vi "Configure Probe.vi"   [LabVIEW 2016, in "Tektronix DPO MSO 2000 4000 Series.lvlib"]
doc: "Select an input type for an oscilloscope and configures the probe settings. The available input types includes:\nAuxiliary Input\nChannel Input"
uses:
  Tektronix DPO MSO 2000 4000 Series.lvlib
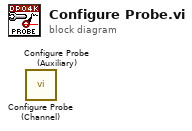
[diagram p0: block diagram]
diagram:
  n1 = call "Configure Probe (Channel).vi"() -> ()  [unwired: 10 in, 2 out]
  n2 = call "Configure Probe (Auxiliary).vi"() -> ()  [unwired: 10 in, 2 out]
